vi "Mouse Move.vi"(8 "error in (no error)":errorcluster, 11 "SwipeScrollListbox in":refnum<class "SwipeScrollListbox.lvclass">) -> (0 "error out":errorcluster, 3 "SwipeScrollListbox out":refnum<class "SwipeScrollListbox.lvclass">)   [LabVIEW 2020, in "SwipeScrollListbox.lvclass"]
uses:
  SwipeScrollListbox.lvclass
  C:/Program Files/National Instruments/LabVIEW 2020/vi.lib/QSI/QControls/QControl Classes/ListBox/ListBox.lvclass
  SwipeScrollListbox.lvclass/SwipeScrollListbox.ctl
  <vilib>/Utility/inputDevices.llb/mouseAcquire.vi
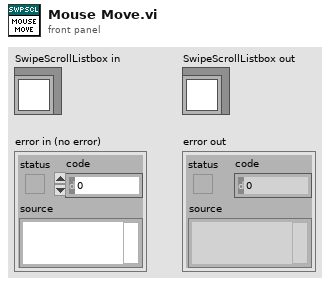
[diagram p1: front panel]
types:
  T1 = typedef "SwipeScrollListbox.lvclass/State Data.ctl" = cluster{"Timeout":i32, "Time":timestamp, "Y":i32, "Slow Distance":i32, "Rate":dbl, "Row Selected":i32}
  T2 = cluster{"Horizontal":i32, "Vertical":i32, "Scrolling":i32}
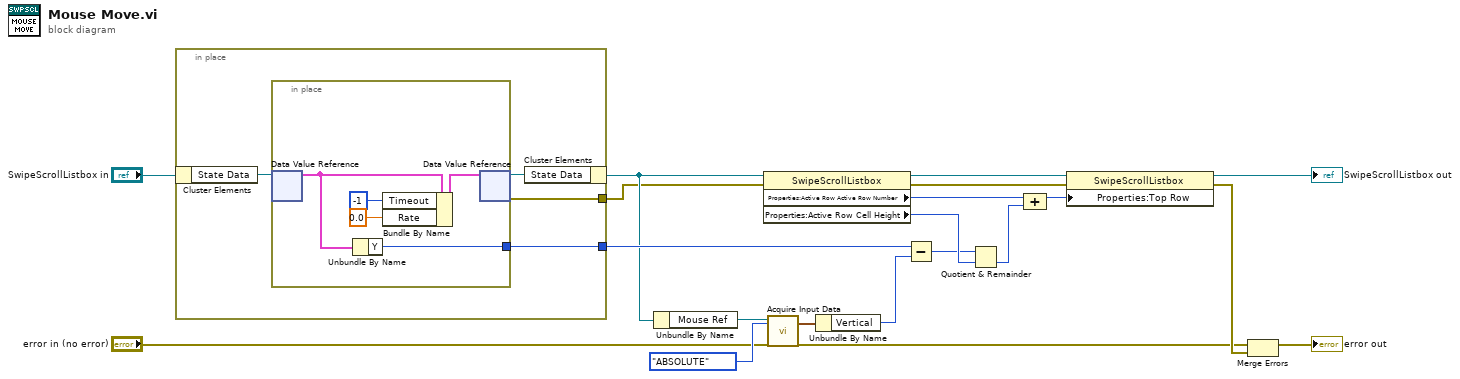
[diagram p0: block diagram]
diagram:
  n1 = in-place {
    in-place-border: [w22] -> w18
    in-place-border: [w21] -> w2
    n2 = in-place-cluster #1("SwipeScrollListbox in") -> ("State Data"=w24:refnum<data-value>)
    n3 = in-place {
      in-place-border: [w25] -> w22
      n4 = in-place-dvr #2(w24) -> (w26:T1)  [unwired: 1 out]
      n5 = Unbundle By Name(w26) -> ("Y"=w25:i32)
      n6 = Bundle By Name(cluster=w26, "Timeout"=-1, "Rate"=0.0) -> (w29:T1)
      n7 = in-place-dvr #2(w29) -> (w23:refnum<data-value>, w21:errorcluster)
    }
    n8 = in-place-cluster #1("State Data"=w23) -> (w3:refnum<class "SwipeScrollListbox.lvclass">)
  }
  n9 = Unbundle By Name(w3) -> ("Mouse Ref"=w15:refnum<k1>)
  n10 = property on="Property Node" class="SwipeScrollListbox"(reference=w3, error in=w2) -> (reference out=w12:refnum<class "SwipeScrollListbox.lvclass">, error out=w11:errorcluster, "Properties:Active Row Active Row Number"=w5:i32, "Properties:Active Row Cell Height"=w13:i32)
  n11 = call-poly <vilib>:"Acquire Input Data.vi"("device ID"=w15, "key mode"=enum16{"RELATIVE", "ABSOLUTE"}."ABSOLUTE", "error in (no error)"="error in (no error)") -> ("axis info"=w14:T2, "error out"=w7:errorcluster)  [unwired: 13 in, 2 out]
  n12 = Unbundle By Name(w14) -> ("Vertical"=w9:i32)
  n13 = Subtract(x=w18, y=w9) -> (x-y=w1:i32)
  n14 = Quotient & Remainder(x=w1, y=w13) -> (floor(x/y)=w6:i32)  [unwired: 1 out]
  n15 = Compound Arithmetic op=ADD(w5, w6) -> (w4:i32)
  n16 = property on="Property Node" class="SwipeScrollListbox"(reference=w12, error in=w11, "Properties:Top Row"=w4) -> (reference out=→"SwipeScrollListbox out":refnum<class "SwipeScrollListbox.lvclass">, error out=w16:errorcluster)
  n17 = Merge Errors(w7, w16) -> (→"error out":errorcluster)
